vi "Start_Sample.vi"(8 "error in (no error)":errorcluster, 10 "SampleList Data":string[](array[string])) -> (0 "error out":errorcluster)   [LabVIEW 2013]
doc: "The input array has all the information for the next analysis (ID, Name, Type) and the run-script.\nWrite the analysis info into a variable and start the script"
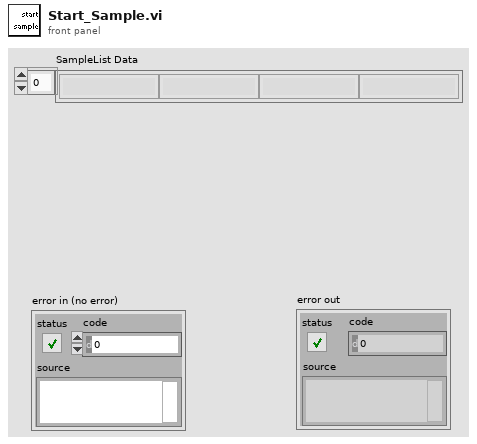
[diagram p1: front panel]
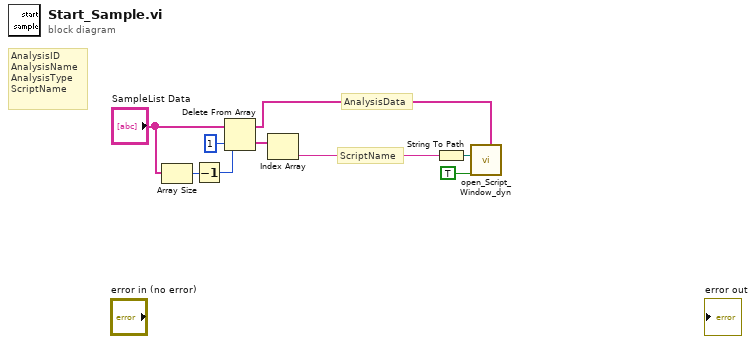
[diagram p0: block diagram]
diagram:
  # "ScriptName"
  # "AnalysisData"
  # "AnalysisID\nAnalysisName\nAnalysisType\nScriptName"
  n1 = Array Size(array="SampleList Data") -> (size(s)=w2:i32)
  n2 = Decrement(x=w2) -> (x-1=w1:i32)
  n3 = Delete From Array(array="SampleList Data", length=1, index=w1) -> (deleted portion=w4:string[], array with subset deleted=w5:string[])
  n4 = Index Array(array=w4) -> (element=w3:string)  [unwired: 1 in]
  n5 = String To Path(string=w3) -> (path=w9:path)
  n6 = call "open_Script_Window_dyn.vi"("AnalysisData"=w5, "run/stop button"=TRUE, "Script Path"=w9) -> ()  [unwired: 8 in, 1 out]
